vi "Write Datalog File.vi"   [LabVIEW 2023]
doc: "Creates a datalog file and writes a specified number of records to the datalog file. Each record is a cluster containing an ID string and an array of numbers."
uses:
  support/Datalog Record.ctl
panel:
  # "Overview: Demonstrates the use of the Datalog functions to write data to a datalog file.\nInstructions:\n1. Run this VI.\n2. Open Read Datalog File.vi and follow the instructions on its front panel."
types:
  T1 = typedef "Datalog Record.ctl" = cluster{"Record ID String":string, "Numeric Data":dbl[]}
  T2 = enum16{"open", "replace", "create", "open or create", "replace or create", "replace or create with confirmation"}
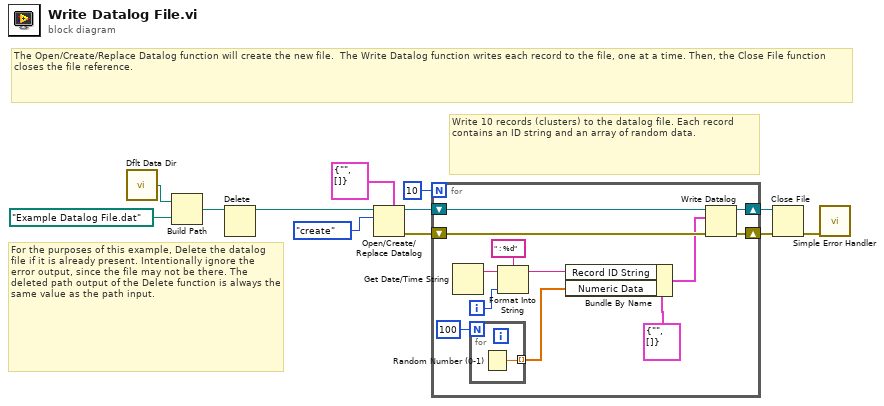
[diagram p0: block diagram]
diagram:
  # "Write 10 records (clusters) to the datalog file. Each record contains an ID string and an array of random data."
  # "The Open/Create/Replace Datalog function will create the new file.  The Write Datalog function writes each record to the file, one at a time. Then, the Close File function closes the file reference."
  # "For the purposes of this example, Delete the datalog file if it is already present. Intentionally ignore the error output, since the file may not be there. The deleted path output of the Delete function is always the same value as the path input."
  n1 = call <vilib>:"Dflt Data Dir.vi"() -> ("App:Default Data Directory"=w4:path)
  n2 = Build Path(base path=w4, name or relative path=path "Example Datalog File.dat" ("default name")) -> (appended path=w2:path)
  n3 = Delete(path (use dialog)=w2) -> (deleted path=w1:path)  [unwired: 4 in, 2 out]
  n4 = Open/Create/Replace Datalog(5:T1 {"Record ID String"="", "Numeric Data"=[]} ("Datalog Record"), 10:T2."create" ("operation (0:open)"), 11:w1) -> (0:w10:errorcluster, 3:w9:refnum<k1>)  [unwired: 1 in, 3 out]
  n5 = for {
    N: 10 ("Number of Acquisitions") -> [_]
    shift-right: [w21] -> w8
    shift-left: w9 -> [w22]
    shift-right: [w24] -> w11
    shift-left: w10 -> [w23]
    i -> [w15]
    n6 = Get Date/Time String() -> (date string=w16:string)  [unwired: 4 out]
    n7 = for {
      N: 100 ("Number of Acquisitions") -> [_]
      tunnel: [w25] -> w20 mode=indexing
      n8 = Random Number (0-1)() -> (number: 0 to 1=w25:dbl)
    }
    n9 = Format Into String(format string=" : %d", initial string=w16, w15) -> (resulting string=w14:string)  [unwired: 1 in, 1 out]
    n10 = Bundle By Name(cluster=T1 {"Record ID String"="", "Numeric Data"=[]} ("Datalog Record"), "Record ID String"=w14, "Numeric Data"=w20) -> (w17:T1)
    n11 = Write Datalog(4:w23, 6:w17, 7:w22) -> (0:w24:errorcluster, 3:w21:refnum<k1>)
  }
  n12 = Close File(refnum=w8, error in=w11) -> (error out=w12:errorcluster)  [unwired: 1 out]
  n13 = call <vilib>:"Simple Error Handler.vi"("error in (no error)"=w12) -> ()  [unwired: 4 in, 5 out]
